vi "_Monitor.vi"() -> ()   [LabVIEW 2017]
uses:
  TagDB/_Support/Multi-Instance/_DEF-DBOper.ctl
  TagDB/TagDB.lvlib
panel:
  out "Count":i32
  in  "Menual Refresh":bool
  in  "Page":enum16{"Common", "Table"}(ring)
  in  "Timeout(ms)":u32=500 min=100 max=60000 step=1
  in  "Auto Refresh?":bool
  in  "DB List":i32(listbox)
  in  "Refresh DB List":bool
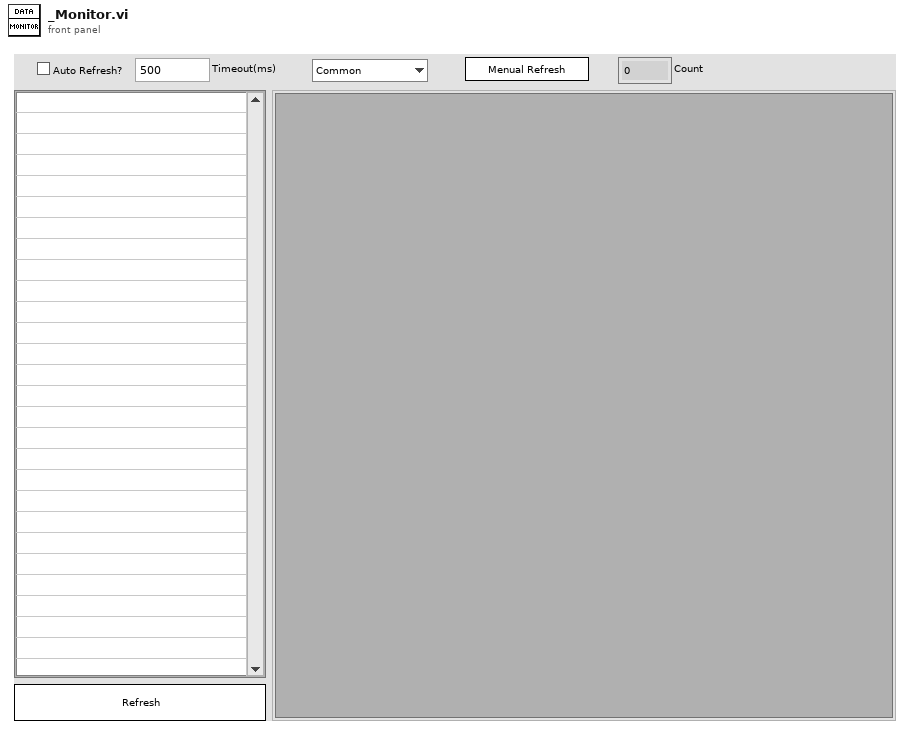
[diagram p1: front panel]
types:
  T1 = cluster{"Sub Panel":refnum<vi>, "DB List":refnum<vi>, "Probe":refnum<vi>, "Tab Probe":refnum<vi>}
  T2 = enum32{"Invalid", "Standard", "Closed", "Hidden", "Minimized", "Maximized"}
  T3 = typedef "TagDB.lvlib/_DEF-DBOper.ctl" = enum16{"create", "destroy", "cleanUp", "list", "get info", "force destroy"}
  T4 = cluster{"DB List":string[], "Page":enum16{"Common", "Table"}}
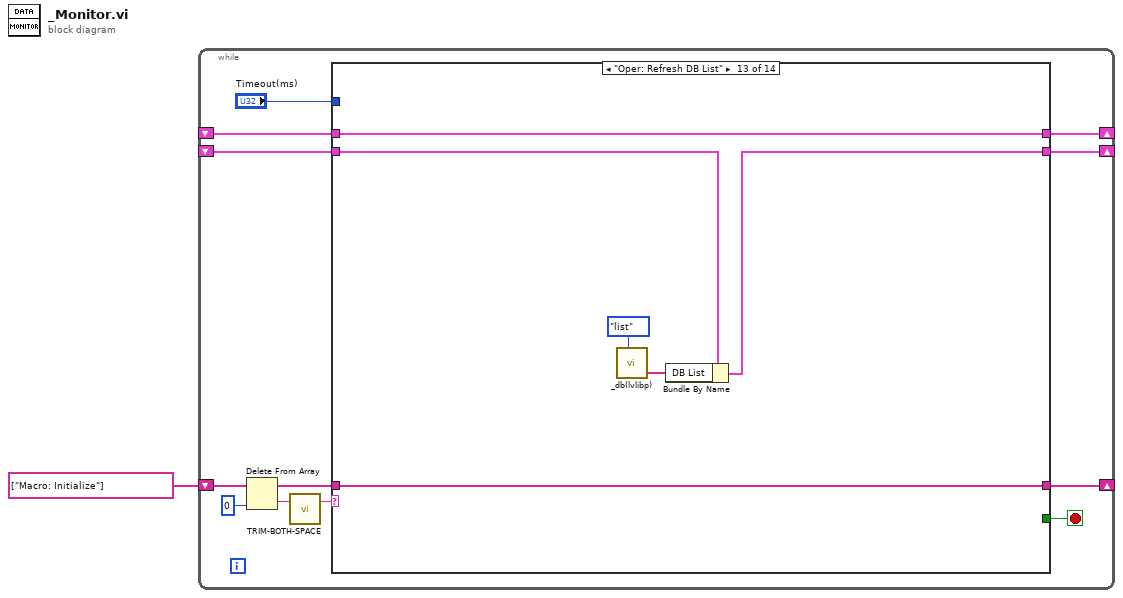
[diagram p0: block diagram]
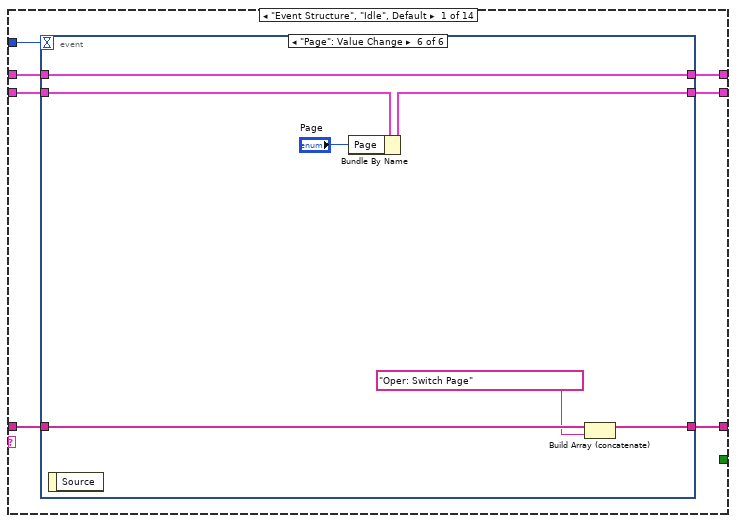
[diagram p2: hidden frame]
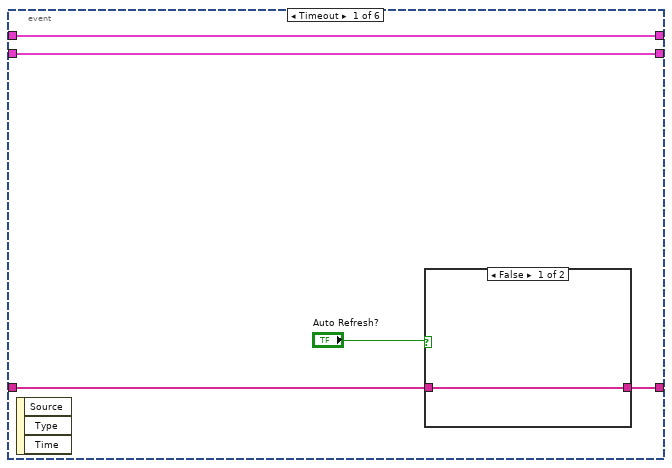
[diagram p3: hidden frame]
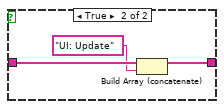
[diagram p4: hidden frame]
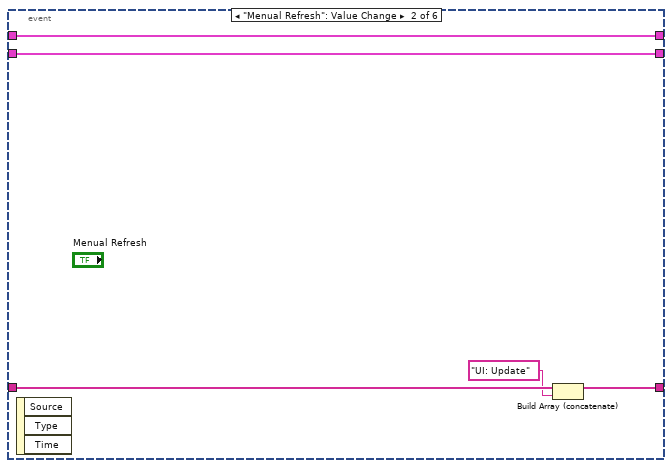
[diagram p5: hidden frame]
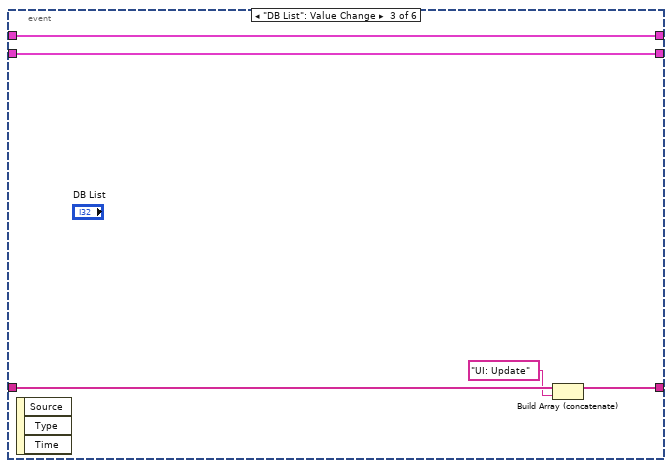
[diagram p6: hidden frame]
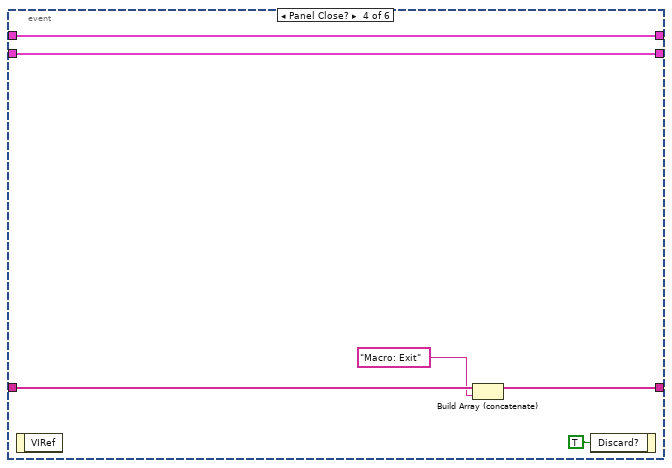
[diagram p7: hidden frame]
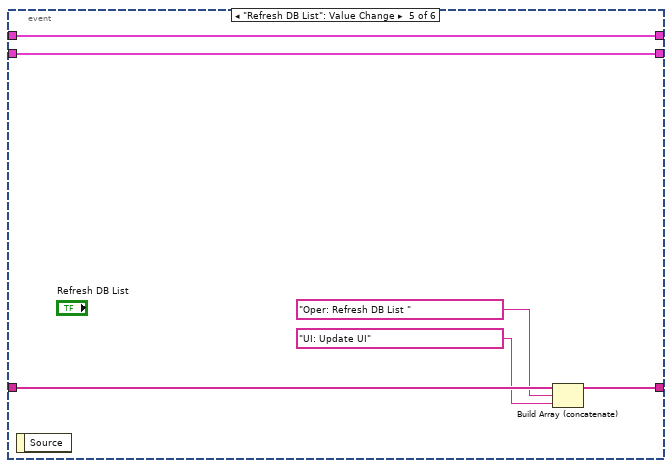
[diagram p8: hidden frame]
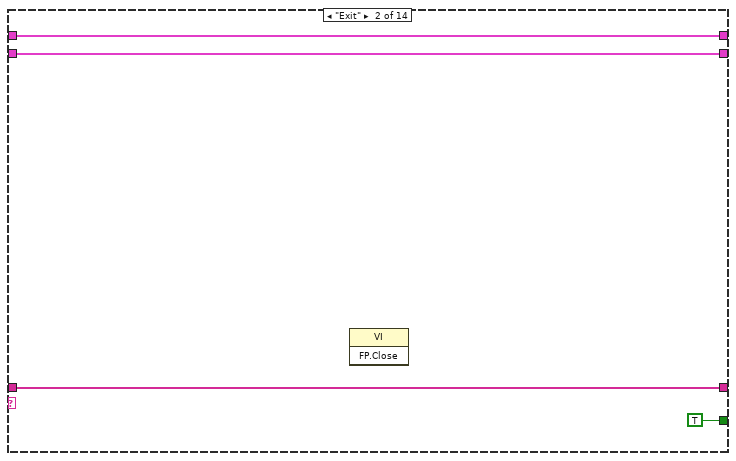
[diagram p9: hidden frame]
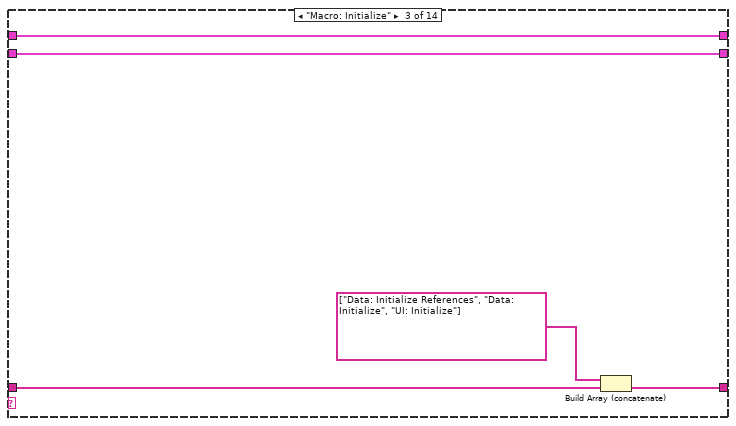
[diagram p10: hidden frame]
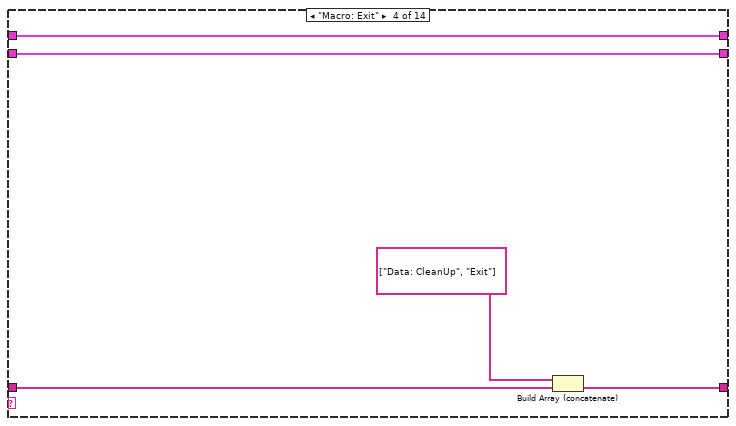
[diagram p11: hidden frame]
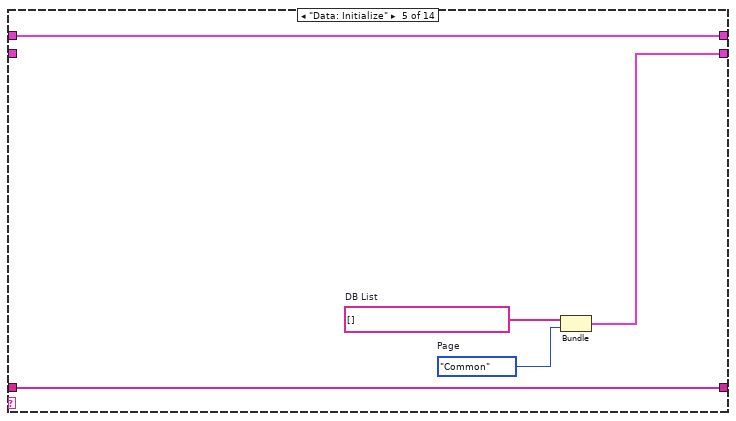
[diagram p12: hidden frame]
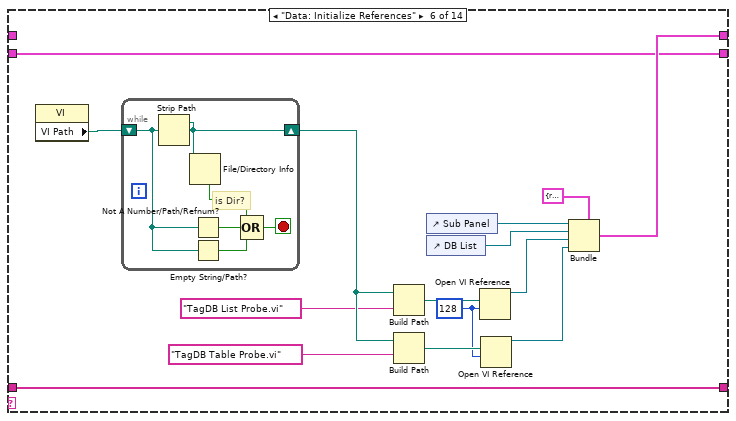
[diagram p13: hidden frame]
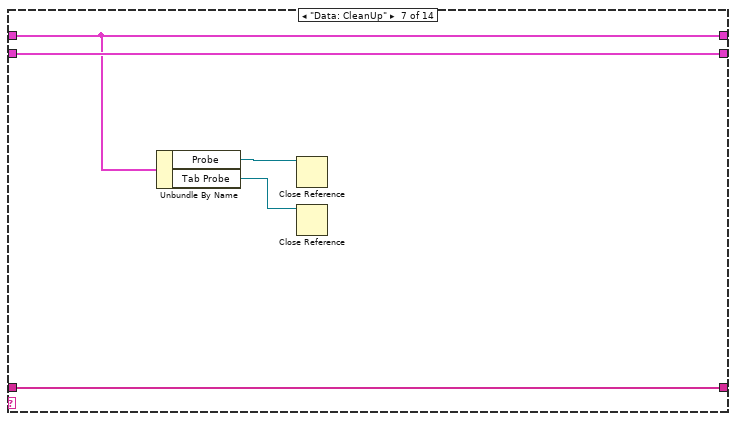
[diagram p14: hidden frame]
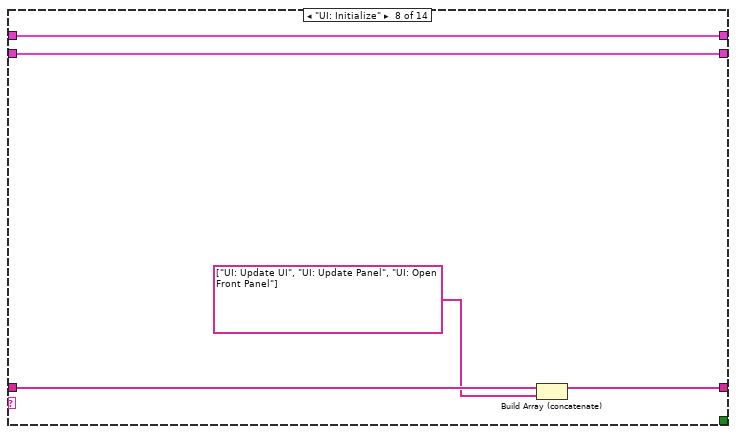
[diagram p15: hidden frame]
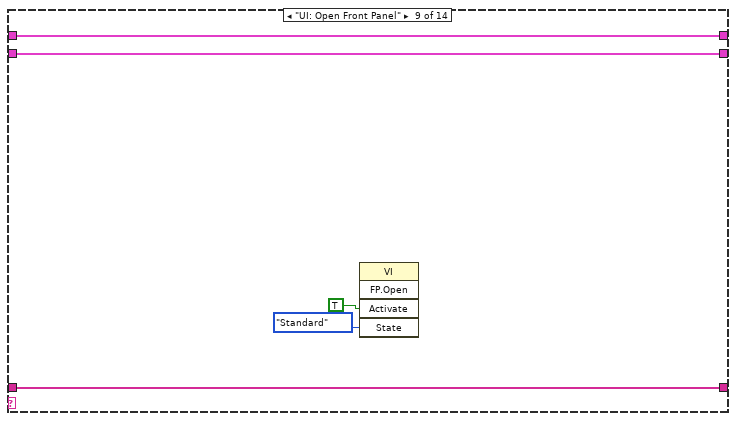
[diagram p16: hidden frame]
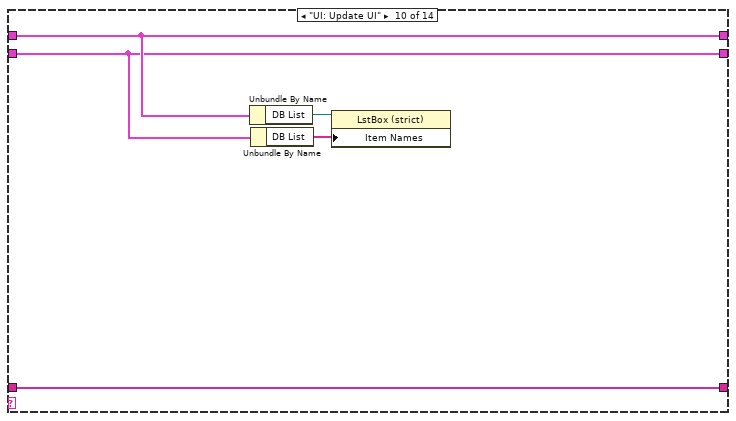
[diagram p17: hidden frame]
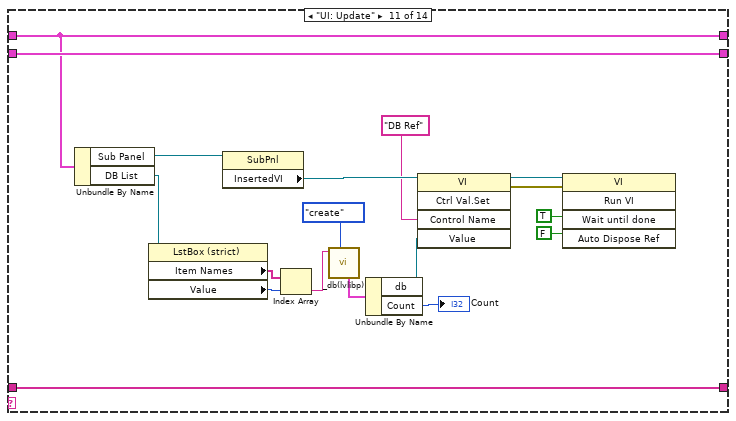
[diagram p18: hidden frame]
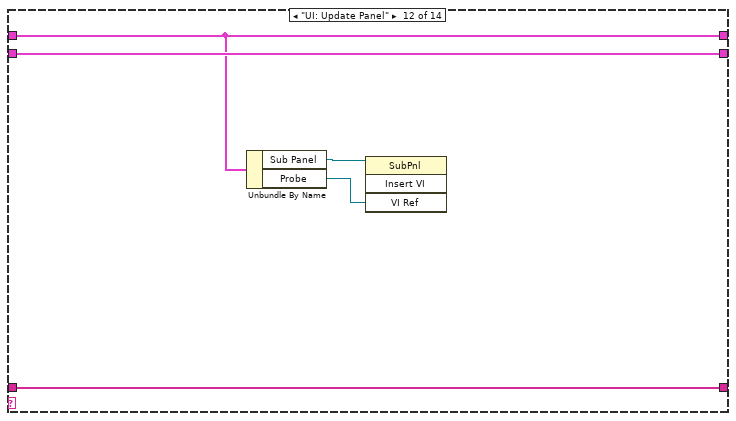
[diagram p19: hidden frame]
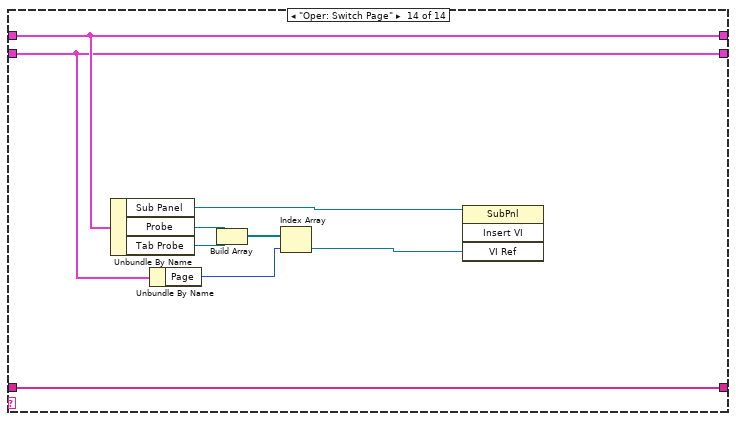
[diagram p20: hidden frame]
diagram:
  n1 = while {
    shift-right: [w8] -> _
    shift-left: string[] ["Macro: Initialize"] -> [w12]
    shift-right: [w7] -> _
    shift-left: _ -> [w6]
    shift-right: [w3] -> _
    shift-left: _ -> [w5]
    stop <- w13 stop-if-true
    n2 = Delete From Array(array=w12, index=0) -> (deleted portion=w11:string, array with subset deleted=w9:string[])  [unwired: 1 in]
    n3 = call "TRIM-BOTH-SPACE.vi"("name in"=w11) -> ("name out"=w4:string)  [unwired: 2 in]
    n4 = case shown="\"Oper: Refresh DB List\"" w4 {
      tunnel: [_ TRUE _ _ _ _ _ _ _ _ _ _ _ _] -> w13
      tunnel: w9 -> [w20 w62 w67 w72 w77 w92 w103 w108 w113 w118 w136 w141 w147 w156]
      tunnel: [w19 w62 w64 w69 w77 w92 w103 w105 w113 w118 w136 w141 w147 w156] -> w8
      tunnel: [w16 w61 w66 w71 w75 w84 w102 w107 w112 w115 w135 w140 w145 w151] -> w7
      tunnel: w6 -> [w15 w61 w66 w71 _ w84 w102 w107 w112 w115 w135 w140 w146 w151]
      tunnel: w5 -> [w17 w60 w65 w70 w73 _ w101 w106 w111 w117 w134 w139 w143 w155]
      tunnel: [w18 w60 w65 w70 w73 w89 w101 w106 w111 w117 w134 w139 w143 w155] -> w3
      tunnel: "Timeout(ms)" -> [w14 _ _ _ _ _ _ _ _ _ _ _ _ _]
      frame "Event Structure", "Idle", Default {
        n5 = event shown="[5] \"Page\": Value Change" {
          selector: _ -> [_ _ _ _ _ _]
          dyn-events: _ -> [_ _ _ _ _ _]
          timeout: w14 -> [_ _ _ _ _ _]
          tunnel: w20 -> [w25 w34 w39 w44 w51 w58]
          tunnel: [w22 w31 w36 w43 w50 w57] -> w19
          tunnel: [w24 w33 w38 w41 w47 w55] -> w18
          tunnel: w17 -> [w24 w33 w38 w41 w47 w55]
          tunnel: [w23 w32 w37 w40 w46 w53] -> w16
          tunnel: w15 -> [w23 w32 w37 w40 w46 w54]
          event Timeout {
            n6 = event-data() -> ()  [unwired: 1 in, 3 out]
            n7 = case shown="False" "Auto Refresh?" {
              tunnel: w25 -> [w26 w29]
              tunnel: [w26 w28] -> w22
              frame False {
              }
              frame True {
                n8 = Build Array (concatenate)(w29, "UI: Update") -> (w28:string[])
              }
            }
          }
          event "Menual Refresh": Value Change {
            n9 = event-data() -> ()  [unwired: 1 in, 3 out]
            n10 = Build Array (concatenate)(w34, "UI: Update") -> (w31:string[])
          }
          event "DB List": Value Change {
            n11 = event-data() -> ()  [unwired: 1 in, 3 out]
            n12 = Build Array (concatenate)(w39, "UI: Update") -> (w36:string[])
          }
          event Panel Close? {
            n13 = event-data() -> ()  [unwired: 1 in, 1 out]
            n14 = Build Array (concatenate)(w44, "Macro: Exit") -> (w43:string[])
            n15 = event-data("Discard?"=TRUE) -> ()  [unwired: 1 in, 1 out]
          }
          event "Refresh DB List": Value Change {
            n16 = event-data() -> ()  [unwired: 1 in, 1 out]
            n17 = Build Array (concatenate)(w51, "Oper: Refresh DB List ", "UI: Update UI") -> (w50:string[])
          }
          event "Page": Value Change {
            n18 = event-data() -> ()  [unwired: 1 in, 1 out]
            n19 = Bundle By Name(cluster=w54, "Page"="Page") -> (w53:T4)
            n20 = Build Array (concatenate)(w58, "Oper: Switch Page") -> (w57:string[])
          }
        }
      }
      frame "Exit" {
        n21 = invoke class="VI" method="FP.Close"() -> ()  [unwired: 3 in, 3 out]
      }
      frame "Macro: Initialize" {
        n22 = Build Array (concatenate)(string[] ["Data: Initialize References", "Data: Initialize", "UI: Initialize"] ("array"), w67) -> (w64:string[])
      }
      frame "Macro: Exit" {
        n23 = Build Array (concatenate)(string[] ["Data: CleanUp", "Exit"] ("array"), w72) -> (w69:string[])
      }
      frame "Data: Initialize" {
        w74 = enum16{"Common", "Table"}."Common"  # Page
        w76 = string[] []  # DB List
        n24 = Bundle("DB List"=w76, "Page"=w74) -> (w75:T4)  [unwired: 1 in]
      }
      frame "Data: Initialize References" {
        w78 = 128 ("options")
        n25 = property class="VI"() -> ("VI Path"=w85:path)  [unwired: 2 in, 2 out]
        n26 = while {
          shift-right: [w93] -> w81
          shift-left: w85 -> [w95]
          stop <- w97 stop-if-true
          # "is Dir?"
          n27 = Strip Path(path=w95) -> (stripped path=w93:path)  [unwired: 1 out]
          n28 = File/Directory Info(path=w93) -> (directory=w98:bool)  [unwired: 1 in, 6 out]
          n29 = Not A Number/Path/Refnum?(number/path/refnum=w95) -> (NaN/Path/Refnum?=w96:bool)
          n30 = Empty String/Path?(string/path=w95) -> (empty?=w94:bool)
          n31 = Compound Arithmetic op=OR(w98, w96, w94) -> (w97:bool)
        }
        n32 = Build Path(base path=w81, name or relative path="TagDB List Probe.vi") -> (appended path=w83:path)
        n33 = Build Path(base path=w81, name or relative path="TagDB Table Probe.vi") -> (appended path=w82:path)
        n34 = control-ref of="Sub Panel"() -> (w91:refnum<vi>)
        n35 = control-ref of="DB List"() -> (w90:refnum<vi>)
        n36 = Open VI Reference(vi path=w83, options=w78) -> (vi reference=w86:refnum<vi>)  [unwired: 4 in, 1 out]
        n37 = Open VI Reference(vi path=w82, options=w78) -> (vi reference=w87:refnum<vi>)  [unwired: 4 in, 1 out]
        n38 = Bundle(cluster=T1 {"Sub Panel"=refnum, "DB List"=refnum, "Probe"=refnum, "Tab Probe"=refnum}, "Sub Panel"=w91, "DB List"=w90, "Probe"=w86, "Tab Probe"=w87) -> (w89:T1)
      }
      frame "Data: CleanUp" {
        n39 = Unbundle By Name(w101) -> ("Probe"=w100:refnum<vi>, "Tab Probe"=w99:refnum<vi>)
        n40 = Close Reference(reference=w100) -> ()  [unwired: 1 in, 1 out]
        n41 = Close Reference(reference=w99) -> ()  [unwired: 1 in, 1 out]
      }
      frame "UI: Initialize" {
        n42 = Build Array (concatenate)(w108, string[] ["UI: Update UI", "UI: Update Panel", "UI: Open Front Panel"] ("array")) -> (w105:string[])
      }
      frame "UI: Open Front Panel" {
        n43 = invoke class="VI" method="FP.Open"("Activate"=TRUE ("Activate?"), "State"=T2."Standard") -> ()  [unwired: 3 in, 5 out]
      }
      frame "UI: Update UI" {
        n44 = Unbundle By Name(w117) -> ("DB List"=w116:refnum<vi>)
        n45 = Unbundle By Name(w115) -> ("DB List"=w114:string[])
        n46 = property class="LstBox (strict)"(reference=w116, "Item Names"=w114) -> ()  [unwired: 1 in, 2 out]
      }
      frame "UI: Update" {
        n47 = Unbundle By Name(w134) -> ("Sub Panel"=w133:refnum<vi>, "DB List"=w131:refnum<vi>)
        n48 = property class="LstBox (strict)"(reference=w131) -> ("Item Names"=w130:string[], "Value"=w129:i32)  [unwired: 1 in, 2 out]
        n49 = property class="SubPnl"(reference=w133) -> ("InsertedVI"=w132:refnum<vi>)  [unwired: 1 in, 2 out]
        n50 = Index Array(array=w130, index=w129) -> (element=w128:string)
        n51 = call "_db(lvlibp).vi"("command"=_DEF-DBOper."create", "name"=w128) -> ("info"=w122:cluster{"db":refnum<k1>, "Count":i32})  [unwired: 5 in, 4 out]
        n52 = Unbundle By Name(w122) -> ("db"=w121:refnum<k1>, "Count"=→"Count":i32)
        n53 = invoke class="VI" method="Ctrl Val.Set"(reference=w132, "Control Name"="DB Ref", "Value"=w121) -> (reference out=w126:refnum<vi>, error out=w125:errorcluster)  [unwired: 2 in, 3 out]
        n54 = invoke class="VI" method="Run VI"(reference=w126, error in=w125, "Wait until done"=TRUE ("Wait Until Done"), "Auto Dispose Ref"=FALSE ("Auto Dispose Reference")) -> ()  [unwired: 1 in, 5 out]
      }
      frame "UI: Update Panel" {
        n55 = Unbundle By Name(w139) -> ("Sub Panel"=w138:refnum<vi>, "Probe"=w137:refnum<vi>)
        n56 = invoke on="Invoke Node" class="SubPnl" method="Insert VI"(reference=w138, "VI Ref"=w137) -> ()  [unwired: 2 in, 4 out]
      }
      frame "Oper: Refresh DB List" {
        n57 = call "_db(lvlibp).vi"("command"=_DEF-DBOper."list") -> ("db list"=w144:string[])  [unwired: 6 in, 4 out]
        n58 = Bundle By Name(cluster=w146, "DB List"=w144) -> (w145:T4)
      }
      frame "Oper: Switch Page" {
        n59 = Unbundle By Name(w155) -> ("Sub Panel"=w149:refnum<vi>, "Probe"=w154:refnum<vi>, "Tab Probe"=w153:refnum<vi>)
        n60 = Unbundle By Name(w151) -> ("Page"=w150:enum16{"Common", "Table"})
        n61 = Build Array(w154, w153) -> (w152:refnum<vi>[])
        n62 = Index Array(array=w152, index=w150) -> (element=w148:refnum<vi>)
        n63 = invoke class="SubPnl" method="Insert VI"(reference=w149, "VI Ref"=w148) -> ()  [unwired: 2 in, 4 out]
      }
    }
  }
